vi "Send Command.vi"() -> (3 "read buffer":string)   [LabVIEW 2020]
uses:
  <vilib>/Instr/_visa.llb/VISA Configure Serial Port (Instr).vi
panel:
  out "substring":string
  out "number 2":dbl format="%.2f"
  out "length 2":i32
  in  "byte":i32
  in  "length (rest)":i32
  out "Numeric":i32
  out "number":dbl format="%.2f"
  out "x+1":i32
  out "Erro 3":bool
  out "length 3":i32
  out "Data field 4":string
  in  "Read":bool
  out "Data field 2":string
  out "Data field":string
  out "Status":string="00570002"
  out "Erro":bool
  in  "No Ack Flag":bool
  in  "Revision of MID":u32
  in  "MID":u32
  in  "Funcao":enum16{"Init", "Message", "End"}(ring)
  out "error out":errorcluster
  in  "data in":string="00200060             "
  in  "Send data":bool
  out "Return Code":i32
  out "length":i32
  out "Complete Data":string="00570002"
  out "data out":string
  in  "Server Closed":string="The server VI closed the connection."
  in  "Stop":bool
  in  "VISA resource name":refnum<visa-resource-name>="COM2"
  # "Alarm Status: 002000700010"
  # "Connection Response\n\nInitial Data: 00570002\nData out:             010000020003"
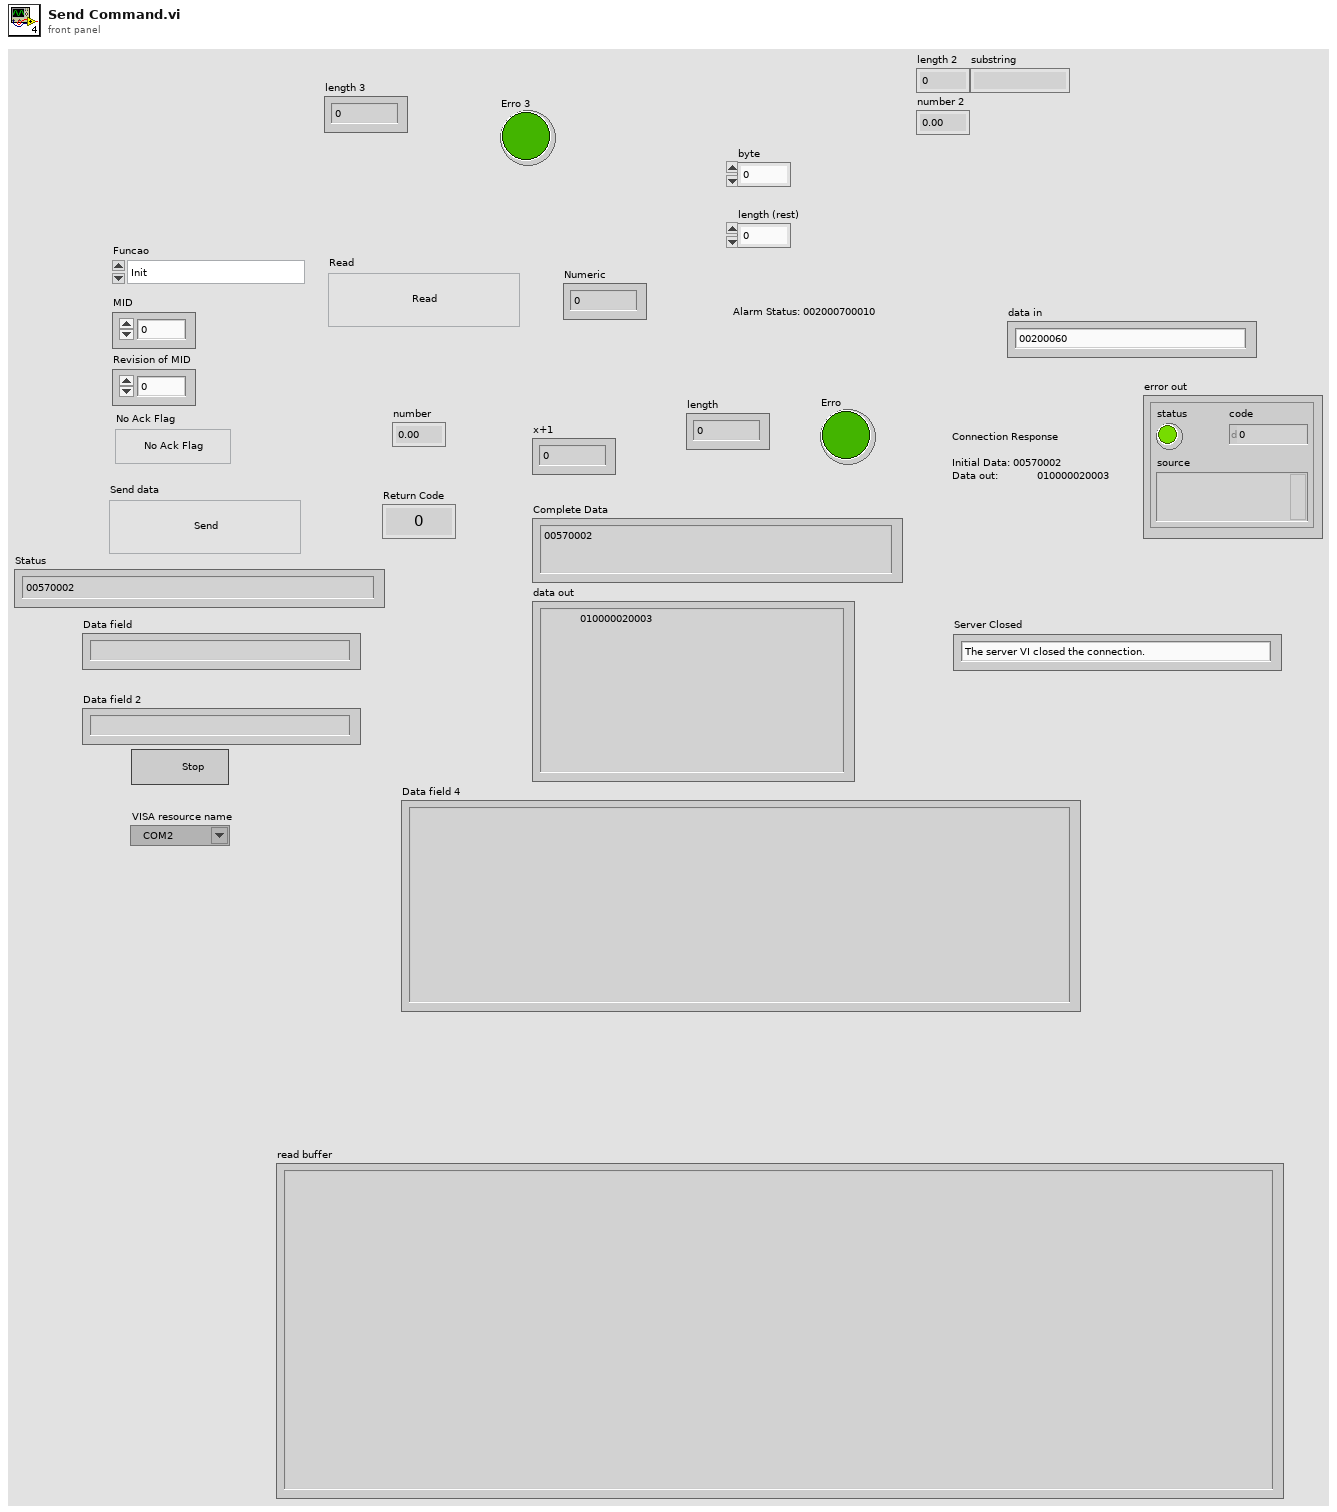
[diagram p1: front panel]
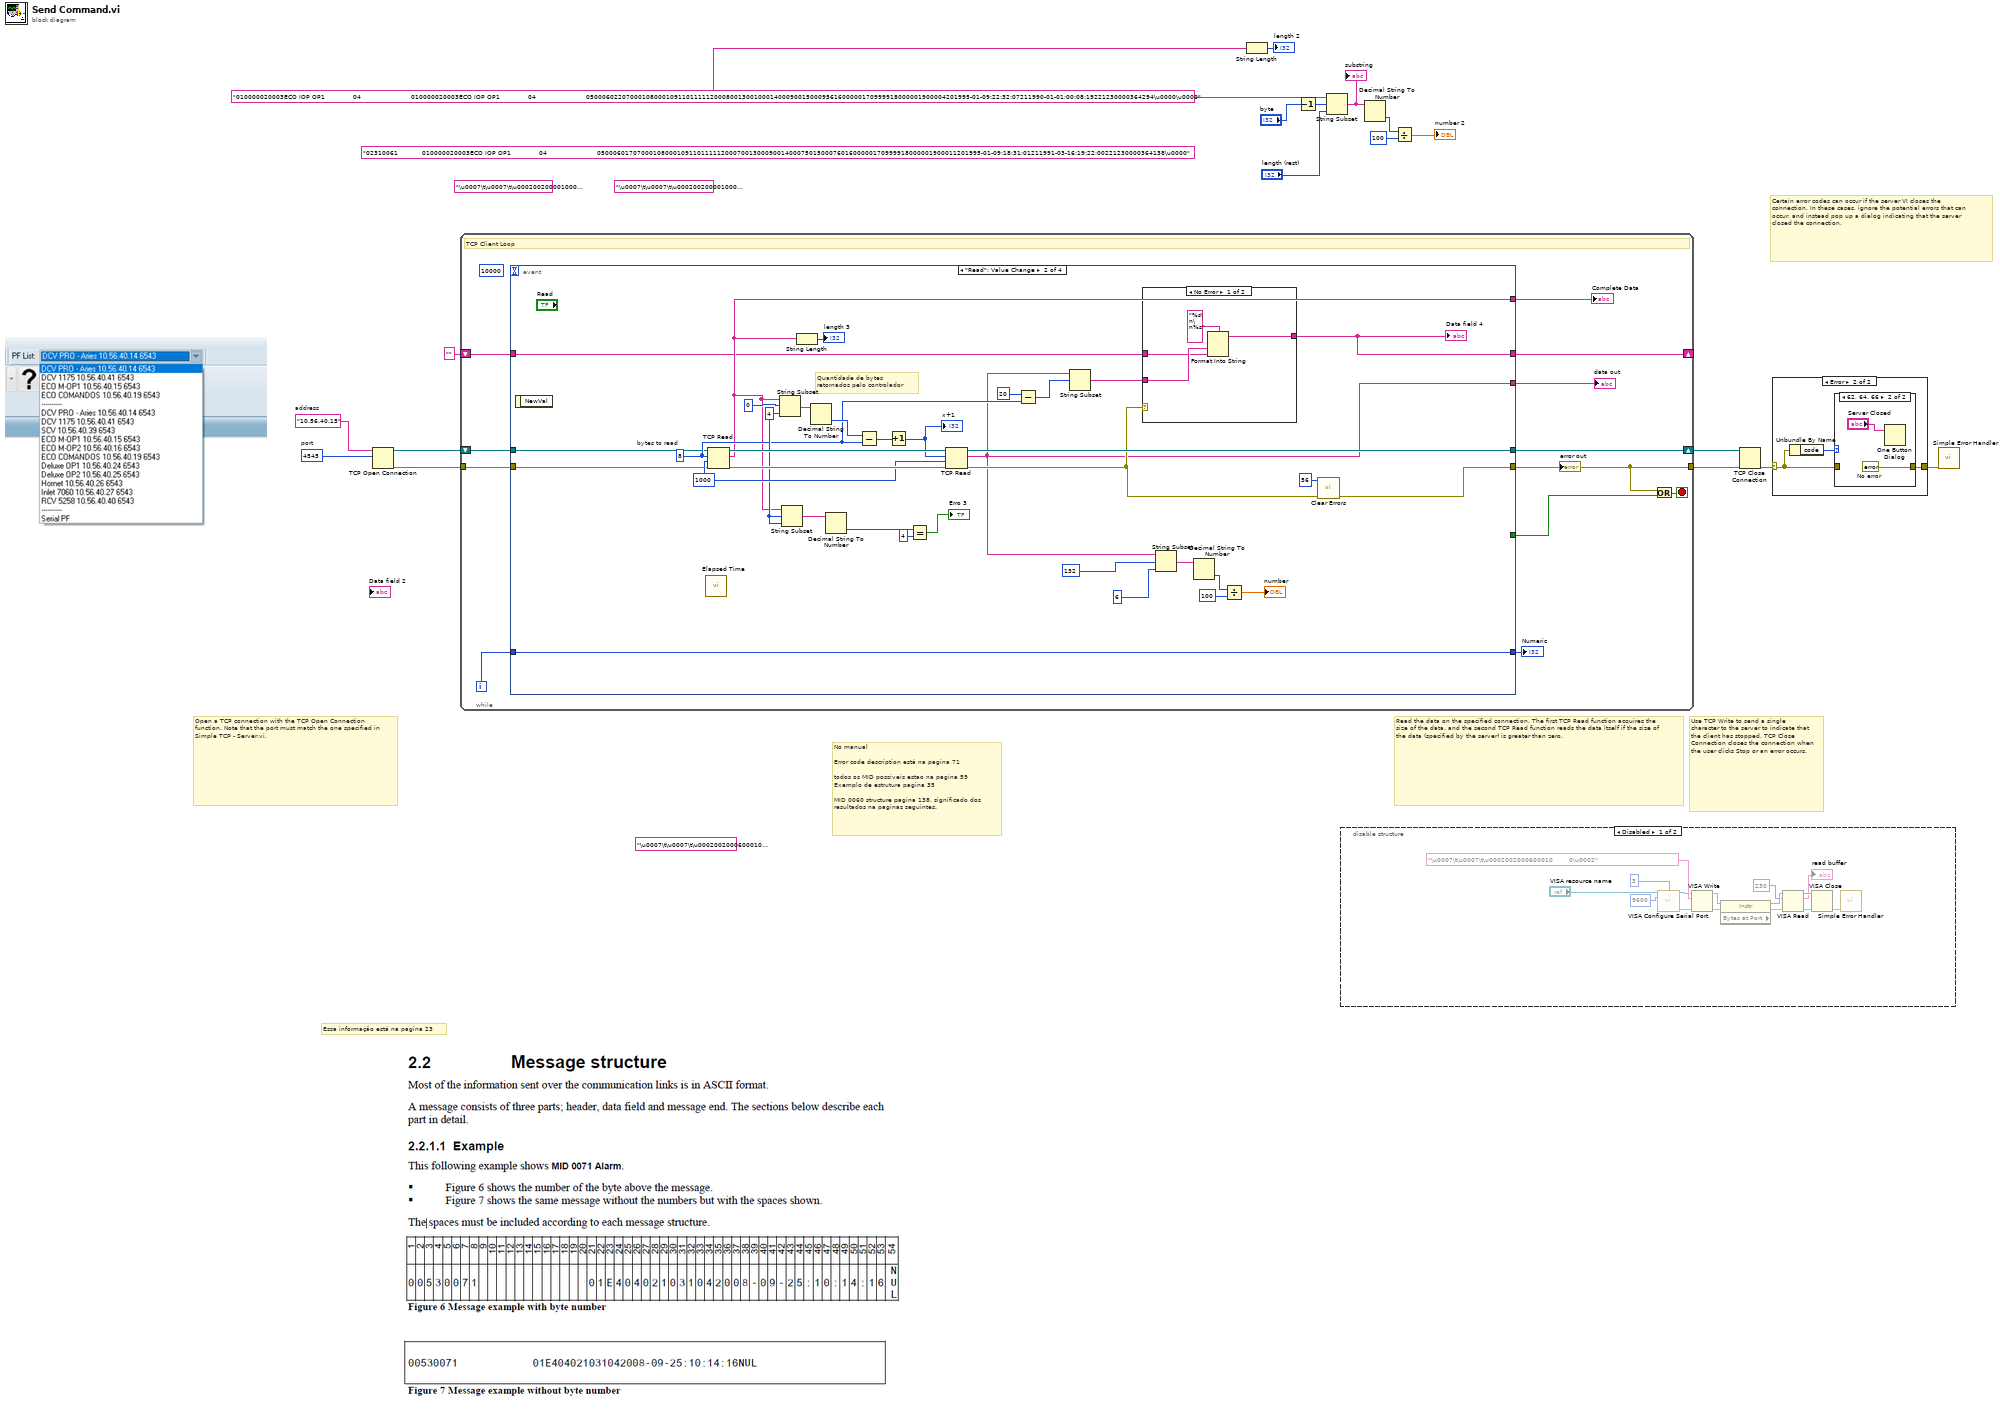
[diagram p0: block diagram]
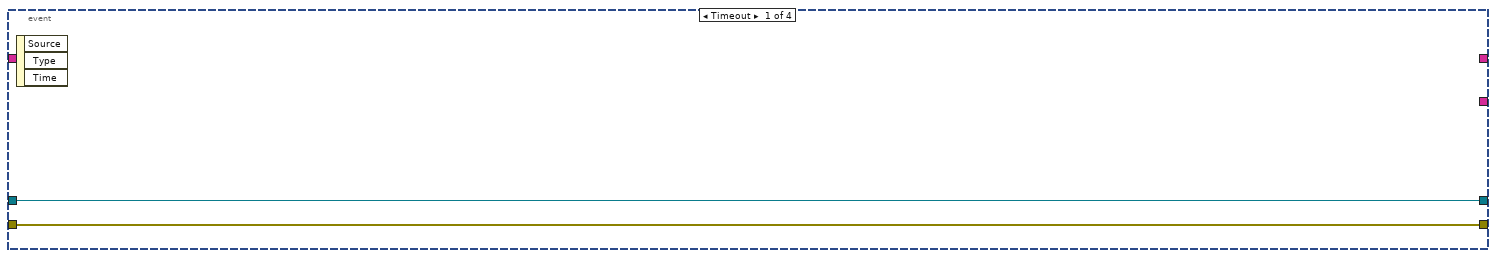
[diagram p2: hidden frame]
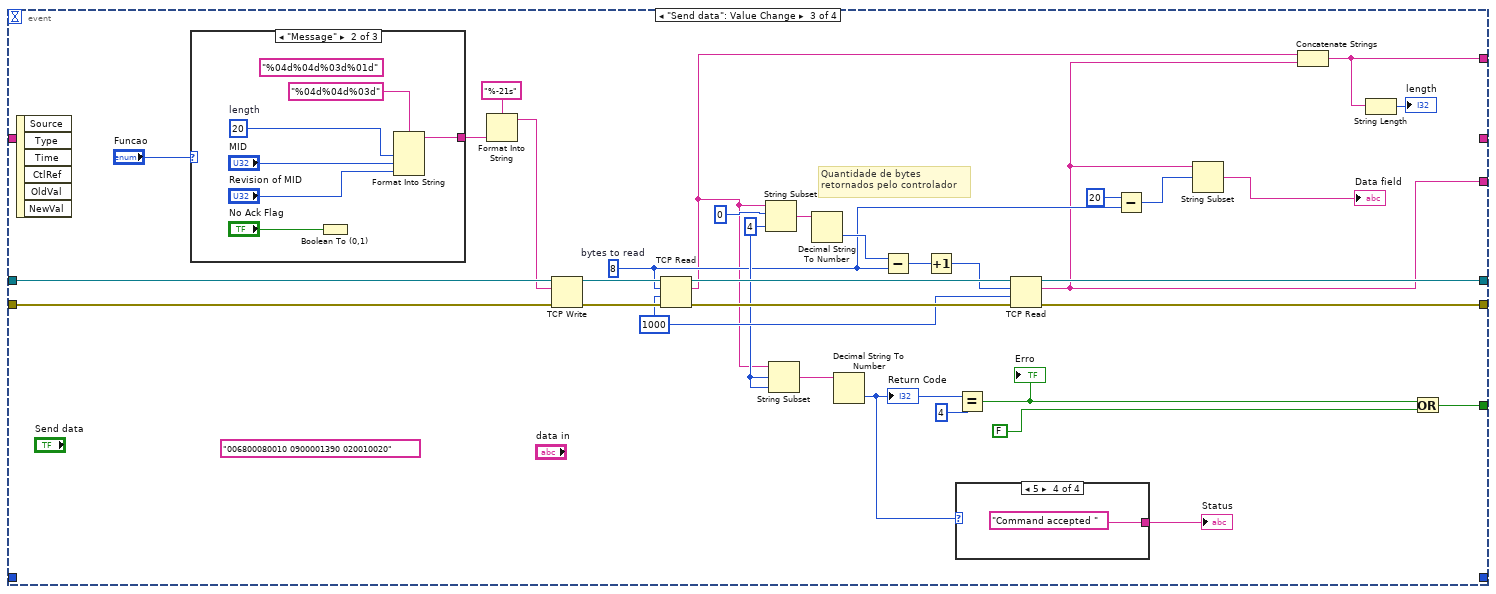
[diagram p4: hidden frame]
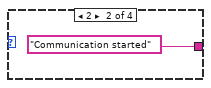
[diagram p6: hidden frame]
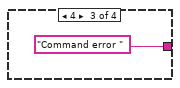
[diagram p7: hidden frame]
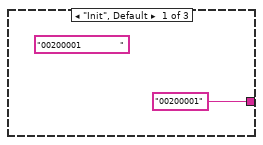
[diagram p8: hidden frame]
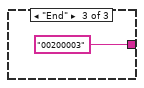
[diagram p9: hidden frame]
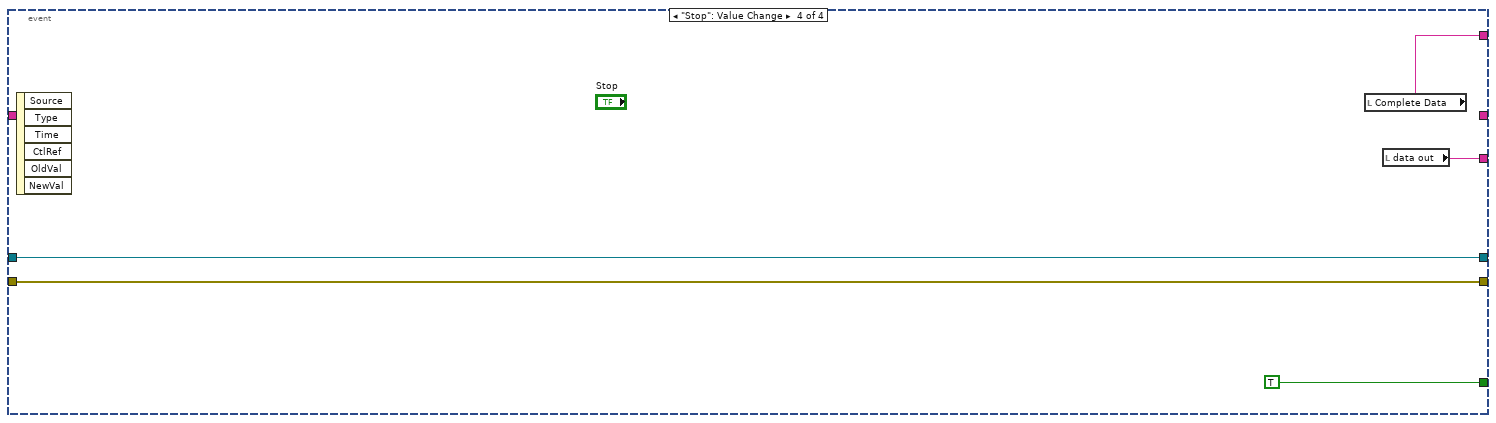
[diagram p10: hidden frame]
diagram:
  (unwired) "02310061            010000020003ECO IOP OP1              04                         050006017070001080001091101111120007001300090014000750150007601600000170999918000001900011201995-01-09:18:31:01211991-03-16:19:22:00221230000364138\u0000" ("string")
  w6 = "010000020003ECO IOP OP1              04                         010000020003ECO IOP OP1              04                         050006022070001080001091101111120008001300100014000900150009561600000170999918000001900004201995-01-09:22:32:07211990-01-01:00:08:19221230000364294\u0000\u0000" ("string")
  (unwired) "\u0007\t\u0007\t\u000200200001000         0\u0003" ("write buffer")
  (unwired) "\u0007\t\u0007\t\u000200200001000         0\u0003" ("write buffer")
  (unwired) "\u0007\t\u0007\t\u0002002000600010        0\u0002" ("write buffer")
  w13 = u16 4545  # port
  w14 = "10.56.40.15"  # address
  # "Essa informação está na pagina 23"
  # "No manual\n\nError code description está na pagina 71\n\ntodos os MID possiveis estao na pagina 59\nExemplo de estrutura pagina 35\n\nMID 0060 structure pagina 138, significado dos\nresultados na paginas seguintes."
  # "Certain error codes can occur if the server VI closes the connection. In these cases, ignore the potential errors that can occur, and instead pop up a dialog indicating that the server closed the connection."
  # "Use TCP Write to send a single character to the server to indicate that the client has stopped. TCP Close Connection closes the connection when the user clicks Stop or an error occurs."
  # "Read the data on the specified connection. The first TCP Read function acquires the size of the data, and the second TCP Read function reads the data itself if the size of the data (specified by the server) is greater than zero."
  # "Open a TCP connection with the TCP Open Connection function. Note that the port must match the one specified in Simple TCP - Server.vi."
  n1 = TCP Open Connection(address=w14, remote port or service name=w13) -> (connection ID=w18:refnum<k5>, error out=w17:errorcluster)  [unwired: 3 in]
  n2 = while {
    tunnel: w17 -> [w29]
    tunnel: [w25] -> w12
    shift-right: [w23] -> w11
    shift-left: w18 -> [w28]
    shift-right: [w22] -> _
    shift-left: "" ("data out") -> [w21]
    i -> [w20]
    stop <- w30 stop-if-true
    (unwired) 10000
    # "TCP Client Loop"
    n3 = event shown="[1] \"Read\": Value Change" {
      selector: _ -> [_ _ _ _]
      dyn-events: _ -> [_ _ _ _]
      timeout: _ -> [_ _ _ _]
      tunnel: w29 -> [w31 w51 w98 w121]
      tunnel: w28 -> [w32 w52 w97 w122]
      tunnel: [_ w35 w73 w118] -> w27
      tunnel: [w32 w50 w96 w122] -> w23
      tunnel: [_ w47 w74 w119] -> w26
      tunnel: [w31 w46 w95 w121] -> w25
      tunnel: [_ _ w87 TRUE] -> w24
      tunnel: [_ w43 _ _] -> w22
      tunnel: w21 -> [_ w42 _ _]
      tunnel: [_ w33 _ _] -> w19
      tunnel: w20 -> [_ w33 _ _]
      event Timeout {
        n4 = event-data() -> ()  [unwired: 1 in, 3 out]
      }
      event "Read": Value Change {
        w60 = 4 ("length (rest)")
        w62 = 1000 ("timeout ms (25000)")
        w55 = 8  # bytes to read
        # "Quantidade de bytes\nretornados pelo controlador"
        n5 = event-data() -> ()  [unwired: 1 in, 1 out]
        n6 = call "Elapsed Time"() -> ()  [unwired: 12 in, 8 out]
        n7 = TCP Read(connection ID=w52, bytes to read=w55, error in (no error)=w51, 9:w62) -> (connection ID out=w64:refnum<k5>, data out=w47:string, error out=w65:errorcluster)  [unwired: 1 in]
        n8 = String Subset(string=w47, offset (0)=0, length (rest)=w60) -> (substring=w66:string)
        n9 = String Subset(string=w47, offset (0)=w60, length (rest)=w60) -> (substring=w61:string)
        n10 = String Length(string=w47) -> (length=→"length 3":i32)
        n11 = Decimal String To Number(string=w66) -> (number=w67:i32)  [unwired: 2 in, 1 out]
        n12 = Decimal String To Number(string=w61) -> (number=w56:i32)  [unwired: 2 in, 1 out]
        n13 = Subtract(x=w67, y=w55) -> (x-y=w59:i32)
        n14 = Increment(x=w59) -> (x+1=w58:i32)
        "x+1" <- w58
        n15 = Equal?(x=w56, y=4) -> (x = y?=→"Erro 3":bool)
        n16 = TCP Read(connection ID=w64, bytes to read=w58, error in (no error)=w65, 9:w62) -> (connection ID out=w50:refnum<k5>, data out=w35:string, error out=w41:errorcluster)  [unwired: 1 in]
        n17 = Subtract(x=20, y=w55) -> (x-y=w53:i32)
        n18 = String Subset(string=w35, offset (0)=w53) -> (substring=w44:string)  [unwired: 1 in]
        n19 = case shown="No Error" w41 {
          tunnel: w44 -> [w70 _]
          tunnel: [w69 w72] -> w43
          tunnel: w42 -> [w68 w72]
          frame No Error {
            n20 = Format Into String(format string="%s\n\n%s", w70, w68) -> (resulting string=w69:string)  [unwired: 2 in, 1 out]
          }
          frame Error {
          }
        }
        "Data field 4" <- w43
        n21 = String Subset(string=w35, offset (0)=132 ("byte"), length (rest)=6 ("length (rest)")) -> (substring=w39:string)
        n22 = Decimal String To Number(string=w39) -> (number=w38:i32)  [unwired: 2 in, 1 out]
        n23 = Divide(x=w38, y=100) -> (x/y=→"number":dbl)
        n24 = call <vilib>:"Clear Errors.vi"("error in (no error)"=w41, "specific error code to clear (0: all)"=56) -> ("error out"=w46:errorcluster)  [unwired: 4 in, 1 out]
      }
      event "Send data": Value Change {
        (unwired) "006800080010 0900001390 020010020" ("write buffer")
        w93 = 4 ("length (rest)")
        w99 = 1000 ("timeout ms (25000)")
        w82 = 8  # bytes to read
        # "Quantidade de bytes\nretornados pelo controlador"
        n25 = event-data() -> ()  [unwired: 1 in, 6 out]
        n26 = case shown="\"Message\"" "Funcao" {
          tunnel: ["00200001" ("data in") w113 "00200003" ("data in")] -> w78
          frame "Init", Default {
            (unwired) "00200001             " ("data in")
          }
          frame "Message" {
            (unwired) "%04d%04d%03d%01d" ("format string")
            w115 = u32 20  # length
            n27 = Boolean To (0,1)(Boolean="No Ack Flag") -> ()  [unwired: 1 out]
            n28 = Format Into String(format string="%04d%04d%03d", w115, "MID", "Revision of MID") -> (resulting string=w113:string)  [unwired: 2 in, 1 out]
          }
          frame "End" {
          }
        }
        n29 = Format Into String(format string="%-21s", w78) -> (resulting string=w77:string)  [unwired: 2 in, 1 out]
        n30 = TCP Write(connection ID=w97, data in=w77, error in (no error)=w98) -> (connection ID out=w102:refnum<k5>, error out=w101:errorcluster)  [unwired: 1 in, 1 out]
        n31 = TCP Read(connection ID=w102, bytes to read=w82, error in (no error)=w101, 9:w99) -> (connection ID out=w103:refnum<k5>, data out=w76:string, error out=w104:errorcluster)  [unwired: 1 in]
        n32 = String Subset(string=w76, offset (0)=0, length (rest)=w93) -> (substring=w105:string)
        n33 = String Subset(string=w76, offset (0)=w93, length (rest)=w93) -> (substring=w94:string)
        n34 = Decimal String To Number(string=w105) -> (number=w106:i32)  [unwired: 2 in, 1 out]
        n35 = Decimal String To Number(string=w94) -> (number=w84:i32)  [unwired: 2 in, 1 out]
        "Return Code" <- w84
        n36 = Subtract(x=w106, y=w82) -> (x-y=w90:i32)
        n37 = Increment(x=w90) -> (x+1=w89:i32)
        n38 = case shown="5" w84 {
          tunnel: [_ "Communication started" ("Status") "Command error " ("Status") "Command accepted " ("Status")] -> w83
          frame 0, Default {
          }
          frame 2 {
          }
          frame 4 {
          }
          frame 5 {
          }
        }
        "Status" <- w83
        n39 = Equal?(x=w84, y=4) -> (x = y?=w88:bool)
        "Erro" <- w88
        n40 = TCP Read(connection ID=w103, bytes to read=w89, error in (no error)=w104, 9:w99) -> (connection ID out=w96:refnum<k5>, data out=w73:string, error out=w95:errorcluster)  [unwired: 1 in]
        n41 = Subtract(x=20, y=w82) -> (x-y=w80:i32)
        n42 = String Subset(string=w73, offset (0)=w80) -> (substring=→"Data field":string)  [unwired: 1 in]
        n43 = Concatenate Strings(w76, w73) -> (w74:string)
        n44 = String Length(string=w74) -> (length=→"length":i32)
        n45 = Or(x=w88, y=FALSE) -> (x .or. y?=w87:bool)
      }
      event "Stop": Value Change {
        n46 = event-data() -> ()  [unwired: 1 in, 6 out]
        n47 = local read "Complete Data"() -> (w119:string)
        n48 = local read "data out"() -> (w118:string)
      }
    }
    "data out" <- w27
    "Complete Data" <- w26
    "error out" <- w25
    "Numeric" <- w19
    n49 = Or(x=w25, y=w24) -> (x .or. y?=w30:bool)
  }
  n50 = String Length(string=w6) -> (length=→"length 2":i32)
  n51 = Decrement(x="byte") -> (x-1=w7:i32)
  n52 = String Subset(string=w6, offset (0)=w7, length (rest)="length (rest)") -> (substring=w4:string)
  "substring" <- w4
  n53 = disable-structure shown="Disabled" {
    frame Disabled {
      n54 = call-poly "VISA Configure Serial Port"("VISA resource name"="VISA resource name", "termination char\n(0xA = '\\n' = LF)"=u8 3 ("termination char\n(0xA = '\\n' = LF)"), "baud rate (9600)"=u32 9600) -> ("VISA resource name out"=w132:refnum<visa-resource-name>, "error out"=w133:errorcluster)  [unwired: 11 in]
      n55 = VISA Write(VISA resource name=w132, write buffer="\u0007\t\u0007\t\u0002002000600010        0\u0002", error in (no error)=w133) -> (VISA resource name out=w125:refnum<visa-resource-name>, error out=w128:errorcluster)  [unwired: 1 out]
      n56 = property class="Instr" props=["Bytes at Port"](reference=w125, error in=w128) -> (reference out=w126:refnum<visa-resource-name>, error out=w127:errorcluster)  [unwired: 1 out]
      n57 = VISA Read(VISA resource name=w126, byte count=u32 230, error in (no error)=w127) -> (VISA resource name out=w136:refnum<visa-resource-name>, read buffer=→"read buffer":string, error out=w137:errorcluster)  [unwired: 1 out]
      n58 = VISA Close(VISA resource name=w136, error in (no error)=w137) -> (error out=w135:errorcluster)
      n59 = call <vilib>:"Simple Error Handler.vi"("error in (no error)"=w135) -> ()  [unwired: 4 in, 5 out]
    }
    frame Enabled {
    }
  }
  n60 = Decimal String To Number(string=w4) -> (number=w3:i32)  [unwired: 2 in, 1 out]
  n61 = Divide(x=w3, y=100) -> (x/y=→"number 2":dbl)
  n62 = TCP Close Connection(connection ID=w11, error in (no error)=w12) -> (error out=w16:errorcluster)  [unwired: 1 in, 1 out]
  n63 = case shown="Error" w16 {
    selector: w16 -> [w138 w140]
    tunnel: [w138 w139] -> w15
    frame No Error {
    }
    frame Error {
      n64 = Unbundle By Name(w140) -> ("code"=w141:i32)
      n65 = case shown="62, 64, 66" w141 {
        tunnel: w140 -> [w142 _]
        tunnel: [w142 w144] -> w139
        frame Default {
        }
        frame 62, 64, 66 {
          w144 = errorcluster {"status"=FALSE, "code"=0, "source"=""}  # No error
          n66 = One Button Dialog(message="Server Closed") -> ()  [unwired: 1 in, 1 out]
        }
      }
    }
  }
  n67 = call <vilib>:"Simple Error Handler.vi"("error in (no error)"=w15) -> ()  [unwired: 4 in, 5 out]
